vi "Parse ERD Read Results.vi"(0 "Converted Data":T4 {"CRC" format="%04x"; "Length" format="%02x"; "Command" format="%02x"; "Destination" format="%02x"; "Source" format="%02x"}, 7 "Read ERD List":T2[](array[typedef]) {"ERD Number" format="%.0x"}) -> (4 "Pass/Fail?":bool, 8 "ERD Data Out":T1[](array[typedef]) {"ERD Number" format="%.0x"})   [LabVIEW 2016, in "GEA2_Toolkit.lvlib"]
doc: "This VI takes the converted return data from the GEA2 Send and Receive and formats the Data based on the selections made in the Read ERD list. In addition, it also verifies the ERDs requested were returned."
uses:
  library/GEA2_Toolkit.lvlib
  type defs/Data Out.ctl
  type defs/ERD Read Data In.ctl
  type defs/Data Type.ctl
  type defs/ERD Read Data Out.ctl
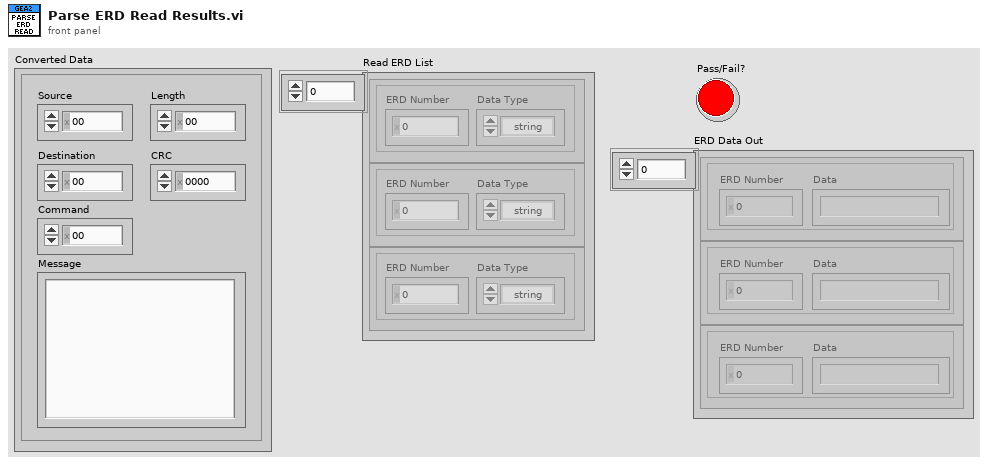
[diagram p1: front panel]
types:
  T1 = typedef "GEA2_Toolkit.lvlib/ERD Read Data Out.ctl" = cluster{"ERD Number":u16, "Data":string}
  T2 = typedef "GEA2_Toolkit.lvlib/ERD Read Data In.ctl" = cluster{"ERD Number":u16, "Data Type":T3}
  T3 = typedef "GEA2_Toolkit.lvlib/Data Type.ctl" = enum16{"string", "boolean", "uint8_t", "uint16_t", "uint32_t", "uint64_t"}
  T4 = typedef "GEA2_Toolkit.lvlib/Data Out.ctl" = cluster{"Source":u8, "Destination":u8, "Command":u8, "Length":u8, "CRC":u16, "Message":string}
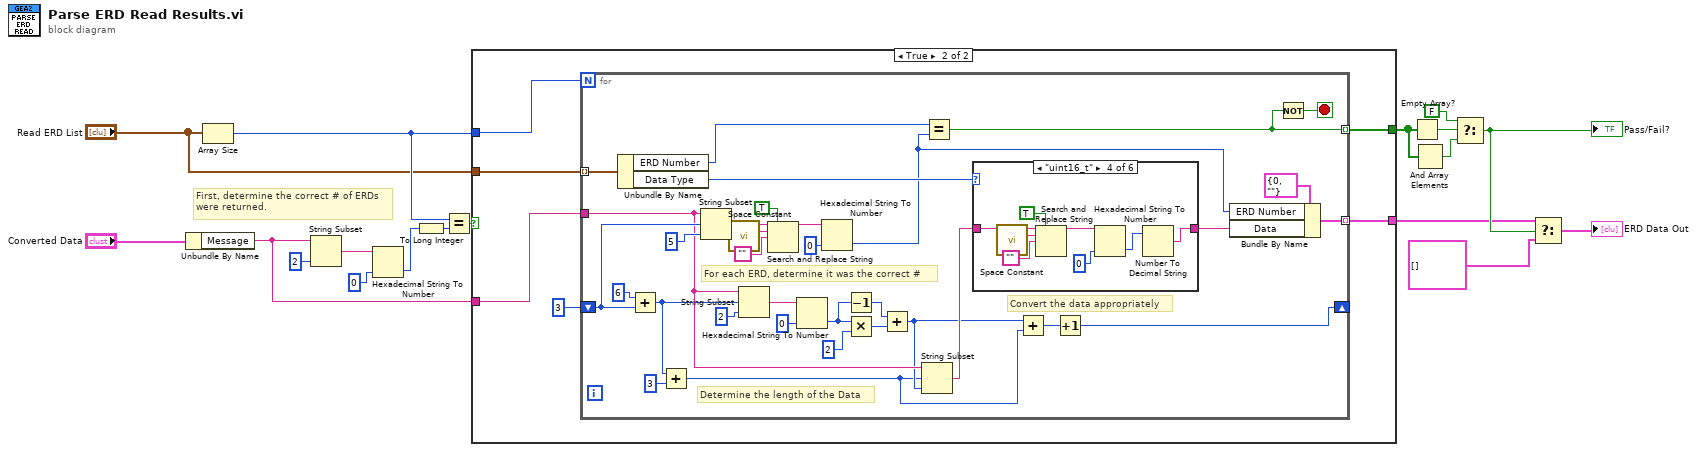
[diagram p0: block diagram]
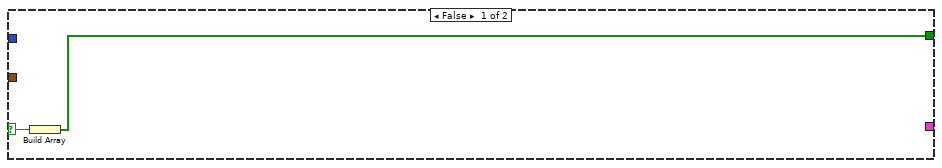
[diagram p2: hidden frame]
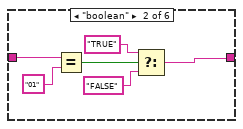
[diagram p4: hidden frame]
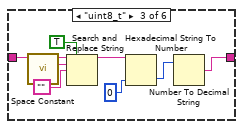
[diagram p5: hidden frame]
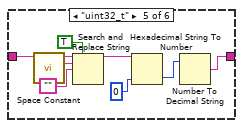
[diagram p6: hidden frame]
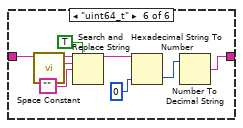
[diagram p7: hidden frame]
diagram:
  # "First, determine the correct # of ERDs\nwere returned."
  n1 = Unbundle By Name("Converted Data") -> ("Message"=w10:string)
  n2 = Array Size(array="Read ERD List") -> (size(s)=w14:i32)
  n3 = String Subset(string=w10, length (rest)=2 ("length (rest)")) -> (substring=w16:string)  [unwired: 1 in]
  n4 = Hexadecimal String To Number(string=w16, default (0uL)=u8 0) -> (number=w12:u8)  [unwired: 1 in, 1 out]
  n5 = To Long Integer(number=w12) -> (32bit integer=w13:i32)
  n6 = Equal?(x=w14, y=w13) -> (x = y?=w11:bool)
  n7 = case shown="True" w11 {
    selector: w11 -> [w20 _]
    tunnel: w14 -> [_ w26]
    tunnel: [w19 w21] -> w8
    tunnel: w10 -> [_ w25]
    tunnel: "Read ERD List" -> [_ w23]
    tunnel: [_ w22] -> w3
    frame False {
      n8 = Build Array(w20) -> (w19:bool[])
    }
    frame True {
      n9 = for {
        N: w26 -> [_]
        tunnel: w25 -> [w49]
        shift-right: [w32] -> _
        shift-left: 3 -> [w53]
        tunnel: w23 -> [w59] mode=indexing
        tunnel: [w38] -> w22 mode=indexing
        tunnel: [w28] -> w21 mode=indexing
        stop <- w29 stop-if-true
        # "Convert the data appropriately"
        # "Determine the length of the Data"
        # "For each ERD, determine it was the correct #"
        n10 = Unbundle By Name(w59) -> ("ERD Number"=w37:u16, "Data Type"=w42:T3)
        n11 = Add(x=6, y=w53) -> (x+y=w48:i32)
        n12 = Add(x=w48, y=3) -> (x+y=w35:i32)
        n13 = String Subset(string=w49, offset (0)=w53, length (rest)=5 ("length (rest)")) -> (substring=w58:string)
        n14 = call <vilib>:"Space Constant.vi"() -> ("String"=w57:string)
        n15 = String Subset(string=w49, offset (0)=w48, length (rest)=2 ("length (rest)")) -> (substring=w51:string)
        n16 = Search and Replace String(replace all?=TRUE ("replace all? (F)"), input string=w58, search string=w57, replace string="") -> (result string=w27:string)  [unwired: 4 in, 3 out]
        n17 = Hexadecimal String To Number(string=w51, default (0uL)=u8 0 ("default (0 U32)")) -> (number=w45:u8)  [unwired: 1 in, 1 out]
        n18 = Hexadecimal String To Number(string=w27, default (0uL)=u16 0) -> (number=w30:u16)  [unwired: 1 in, 1 out]
        n19 = Decrement(x=w45) -> (x-1=w43:u8)
        n20 = Multiply(x=w45, y=u8 2) -> (x*y=w44:u8)
        n21 = Add(x=w43, y=w44) -> (x+y=w36:u8)
        n22 = String Subset(string=w49, offset (0)=w35, length (rest)=w36) -> (substring=w41:string)
        n23 = Equal?(x=w37, y=w30) -> (x = y?=w28:bool)
        n24 = case shown="\"uint16_t\"" w42 {
          tunnel: w41 -> [w60 w66 w72 w78 w86 w94]
          tunnel: [w60 w61 w69 w77 w85 w93] -> w39
          frame "string", Default {
          }
          frame "boolean" {
            n25 = Equal?(x=w66, y="01") -> (x = y?=w64:bool)
            n26 = Select(t="TRUE", s=w64, f="FALSE") -> (s? t:f=w61:string)
          }
          frame "uint8_t" {
            n27 = call <vilib>:"Space Constant.vi"() -> ("String"=w74:string)
            n28 = Search and Replace String(replace all?=TRUE ("replace all? (F)"), input string=w72, search string=w74, replace string="") -> (result string=w71:string)  [unwired: 4 in, 3 out]
            n29 = Hexadecimal String To Number(string=w71, default (0uL)=u8 0) -> (number=w67:u8)  [unwired: 1 in, 1 out]
            n30 = Number To Decimal String(number=w67) -> (decimal integer string=w69:string)  [unwired: 1 in]
          }
          frame "uint16_t" {
            n31 = call <vilib>:"Space Constant.vi"() -> ("String"=w82:string)
            n32 = Search and Replace String(replace all?=TRUE ("replace all? (F)"), input string=w78, search string=w82, replace string="") -> (result string=w80:string)  [unwired: 4 in, 3 out]
            n33 = Hexadecimal String To Number(string=w80, default (0uL)=u16 0) -> (number=w75:u16)  [unwired: 1 in, 1 out]
            n34 = Number To Decimal String(number=w75) -> (decimal integer string=w77:string)  [unwired: 1 in]
          }
          frame "uint32_t" {
            n35 = call <vilib>:"Space Constant.vi"() -> ("String"=w90:string)
            n36 = Search and Replace String(replace all?=TRUE ("replace all? (F)"), input string=w86, search string=w90, replace string="") -> (result string=w88:string)  [unwired: 4 in, 3 out]
            n37 = Hexadecimal String To Number(string=w88, default (0uL)=u32 0) -> (number=w83:u32)  [unwired: 1 in, 1 out]
            n38 = Number To Decimal String(number=w83) -> (decimal integer string=w85:string)  [unwired: 1 in]
          }
          frame "uint64_t" {
            n39 = call <vilib>:"Space Constant.vi"() -> ("String"=w98:string)
            n40 = Search and Replace String(replace all?=TRUE ("replace all? (F)"), input string=w94, search string=w98, replace string="") -> (result string=w96:string)  [unwired: 4 in, 3 out]
            n41 = Hexadecimal String To Number(string=w96, default (0uL)=u64 0) -> (number=w91:u64)  [unwired: 1 in, 1 out]
            n42 = Number To Decimal String(number=w91) -> (decimal integer string=w93:string)  [unwired: 1 in]
          }
        }
        n43 = Add(x=w36, y=w35) -> (x+y=w33:i32)
        n44 = Increment(x=w33) -> (x+1=w32:i32)
        n45 = Bundle By Name(cluster=T1 {"ERD Number"=0, "Data"=""} ("ERD Output"), "ERD Number"=w30, "Data"=w39) -> (w38:T1)
        n46 = Not(x=w28) -> (.not. x?=w29:bool)
      }
    }
  }
  n47 = Empty Array?(array=w8) -> (empty?=w7:bool)
  n48 = And Array Elements(Boolean array=w8) -> (logical AND=w6:bool)
  n49 = Select(t=FALSE, s=w7, f=w6) -> (s? t:f=w4:bool)
  "Pass/Fail?" <- w4
  n50 = Select(t=w3, s=w4, f=T1[] []) -> (s? t:f=→"ERD Data Out":T1[])
